vi "Waveform Generator Output Single Cycle.vi"(0 "VISA resource name":refnum<visa-resource-name>, 5 "Waveform Generator Number (1: Waveform Generator 1)":i32(ring)=1 items=["Waveform Generator 1"=1, "Waveform Generator 2"=2], 11 "error in (no error)":errorcluster) -> (4 "VISA resource name out":refnum<visa-resource-name>, 15 "error out":errorcluster)   [LabVIEW 2016, in "Agilent 2000 3000 X-Series.lvlib"]
doc: "When the single-shot output mode is selected this causes a single cycle of the defined waveform to be output."
uses:
  Agilent 2000 3000 X-Series.lvlib
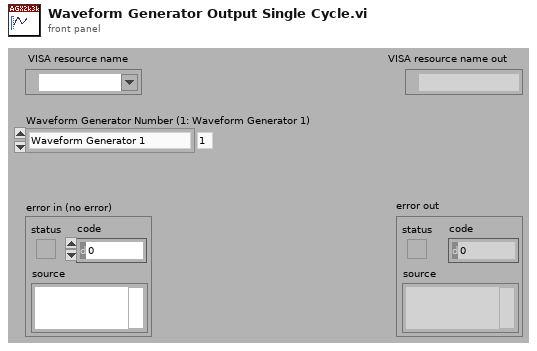
[diagram p1: front panel]
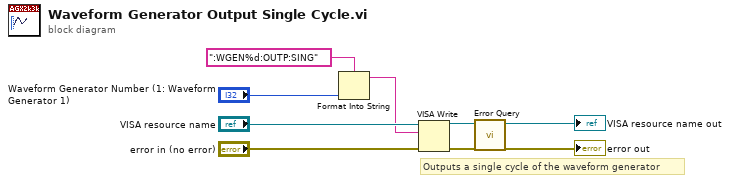
[diagram p0: block diagram]
diagram:
  # "Outputs a single cycle of the waveform generator"
  n1 = Format Into String(format string=":WGEN%d:OUTP:SING", "Waveform Generator Number (1: Waveform Generator 1)") -> (resulting string=w4:string)  [unwired: 2 in, 1 out]
  n2 = VISA Write(VISA resource name="VISA resource name", write buffer=w4, error in (no error)="error in (no error)") -> (VISA resource name out=w2:refnum<visa-resource-name>, error out=w1:errorcluster)  [unwired: 1 out]
  n3 = call "Error Query.vi"("error in (no error)"=w1, "VISA resource name"=w2) -> ("error out"=→"error out":errorcluster, "VISA resource name out"=→"VISA resource name out":refnum<visa-resource-name>)  [unwired: 8 out]
